vi "Configure Sequence Characteristics.vi"(0 "VISA resource name":refnum<visa-resource-name>, 1 "Sequence Step Shape (1: Pulse)":i32(ring)=1 items=["Exponential", "Pulse", "Ramp", "Sine Wave", "Staircase", "Step", "Trapezoid", "User Defined"], 3 "Sequence Step Number (0)":i32, 5 "Channel Name (1)":string="1", 7 "Sequence Step Pacing (1: Dwell)":i32(ring)=1 items=["Triggered", "Dwell"], 9 "Sequence Step Repeat Count (1)":i32=1, 11 "error in (no error)":errorcluster {"code" format="%.0x"}, 12 "Sequence Repeat Count (1)":i32=1, 13 "Sequence Last Termination (False)":bool) -> (4 "VISA resource name out":refnum<visa-resource-name>, 15 "error out":errorcluster {"code" format="%.0x"})   [LabVIEW 2016, in "Agilent N6700 Series.lvlib"]
doc: "Sets the shape, pacing, step number, step repeat count, the sequence repeat count and the output value when the sequence terminates.\n\n<b>Note:</b>\nThis VI only applies to the N6705B and N6705C DC Power Analyzer."
uses:
  <instrlib>/Agilent N6700 Series/Agilent N6700 Series.lvlib
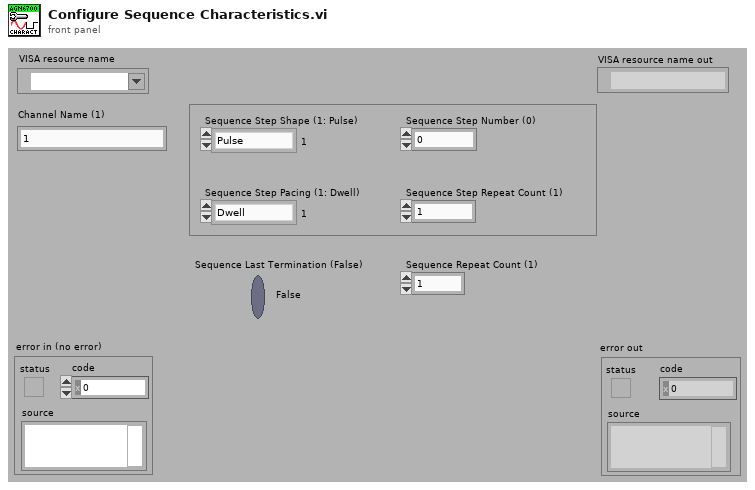
[diagram p1: front panel]
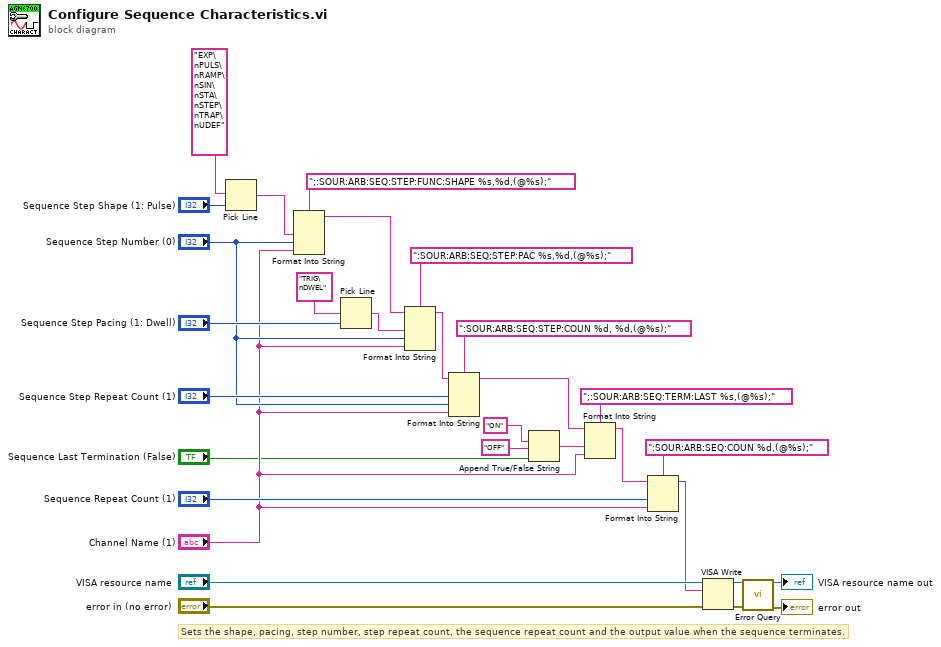
[diagram p0: block diagram]
diagram:
  # "Sets the shape, pacing, step number, step repeat count, the sequence repeat count and the output value when the sequence terminates."
  n1 = Pick Line(multi-line string="EXP\nPULS\nRAMP\nSIN\nSTA\nSTEP\nTRAP\nUDEF" ("string (\"\")"), line index="Sequence Step Shape (1: Pulse)") -> (output string=w23:string)  [unwired: 1 in]
  n2 = Format Into String(format string=";:SOUR:ARB:SEQ:STEP:FUNC:SHAPE %s,%d,(@%s);", w23, "Sequence Step Number (0)", "Channel Name (1)") -> (resulting string=w14:string)  [unwired: 2 in, 1 out]
  n3 = Pick Line(multi-line string="TRIG\nDWEL", line index="Sequence Step Pacing (1: Dwell)") -> (output string=w15:string)  [unwired: 1 in]
  n4 = Format Into String(format string=":SOUR:ARB:SEQ:STEP:PAC %s,%d,(@%s);", initial string=w14, w15, "Sequence Step Number (0)", "Channel Name (1)") -> (resulting string=w12:string)  [unwired: 1 in, 1 out]
  n5 = Format Into String(format string=":SOUR:ARB:SEQ:STEP:COUN %d, %d,(@%s);", initial string=w12, "Sequence Step Repeat Count (1)", "Sequence Step Number (0)", "Channel Name (1)") -> (resulting string=w6:string)  [unwired: 1 in, 1 out]
  n6 = Append True/False String(1:"Sequence Last Termination (False)", 2:"OFF", 3:"ON") -> (0:w9:string)  [unwired: 1 in]
  n7 = Format Into String(format string=";:SOUR:ARB:SEQ:TERM:LAST %s,(@%s);", initial string=w6, w9, "Channel Name (1)") -> (resulting string=w11:string)  [unwired: 1 in, 1 out]
  n8 = Format Into String(format string=":SOUR:ARB:SEQ:COUN %d,(@%s);", initial string=w11, "Sequence Repeat Count (1)", "Channel Name (1)") -> (resulting string=w2:string)  [unwired: 1 in, 1 out]
  n9 = VISA Write(VISA resource name="VISA resource name", write buffer=w2, error in (no error)="error in (no error)") -> (VISA resource name out=w26:refnum<visa-resource-name>, error out=w25:errorcluster)  [unwired: 1 out]
  n10 = call <instrlib>:"Error Query.vi"("VISA resource name"=w26, "error in (no error)"=w25) -> ("VISA resource name out"=→"VISA resource name out":refnum<visa-resource-name>, "error out"=→"error out":errorcluster)  [unwired: 10 in, 2 out]
